vi "max data.vi"() -> (2 "MAX ID":string)   [LabVIEW 2013]
uses:
  <vilib>/addons/database/Connection.llb/DB Tools Open Connec (String).vi
  <vilib>/addons/database/Connection.llb/Conn Execute.vi
  <vilib>/addons/database/Recordset.llb/Rec Fetch Recordset Data (R).vi
  <vilib>/addons/database/Recordset.llb/Rec Destroy - Connection.vi
  <vilib>/addons/database/NI_Database_API.lvlib
panel:
  out "data":string[][](array[string])
  out "recordset data":variant[][](array[variant])
  out "连接的字符串":string
  in  "error in (no error)":errorcluster
  out "error out":errorcluster
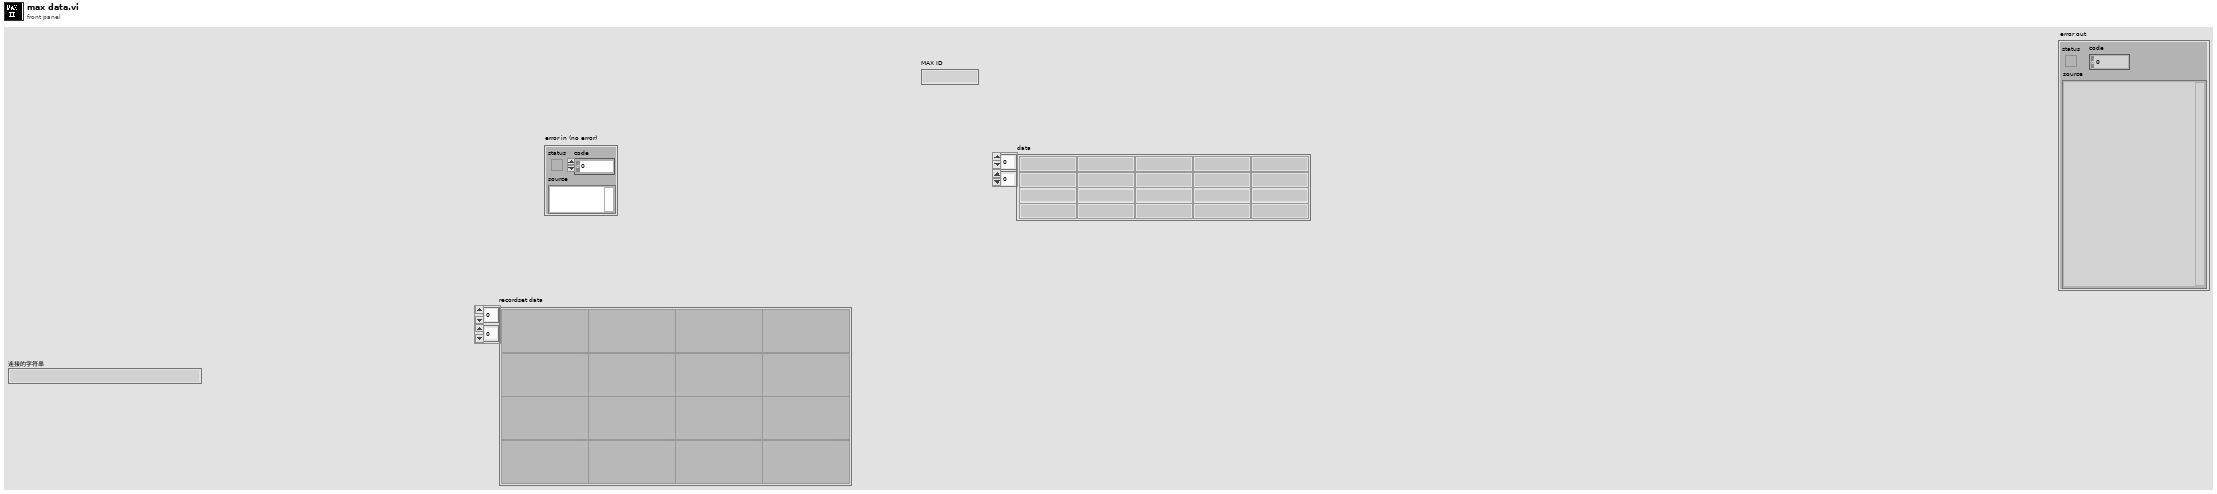
[diagram p1: front panel]
types:
  T1 = typedef "NI_Database_API.lvlib/Conn ObjectReference.ctl" = refnum<k1>
  T2 = typedef "NI_Database_API.lvlib/Rec ObjectReference.ctl" = refnum<k1>
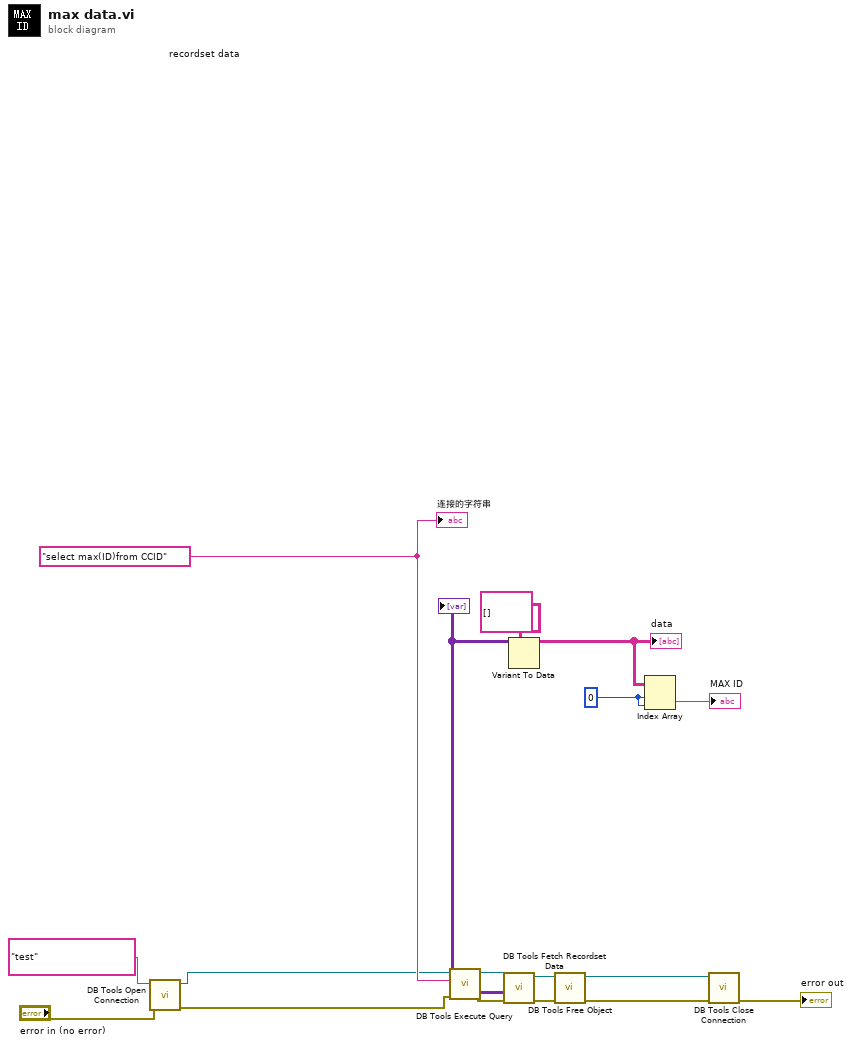
[diagram p0: block diagram]
diagram:
  w2 = 0 ("索引 (行)")
  w6 = "select max(ID)from CCID" ("字符串")
  n1 = call-poly <vilib>:"DB Tools Open Connection.vi"("error in (no error)"="error in (no error)", "connection information"="test" ("userID")) -> ("error out"=w4:errorcluster, "connection reference"=w5:T1)  [unwired: 6 in]
  n2 = call-poly <vilib>:"DB Tools Execute Query.vi"("error in (no error)"=w4, "SQL query"=w6, "connection reference"=w5) -> ("error out"=w14:errorcluster, "recordset reference"=w15:T2)  [unwired: 5 in]
  n3 = call-poly <vilib>:"DB Tools Fetch Recordset Data.vi"("error in (no error)"=w14, "recordset reference"=w15) -> ("error out"=w13:errorcluster, "recordset data"=w10:variant[][], "recordset reference out"=w12:T2)  [unwired: 3 in]
  "recordset data" <- w10
  n4 = Variant To Data(type=string[][] [] ("数组"), Variant=w10) -> (data=w3:string[][])  [unwired: 1 in, 1 out]
  "data" <- w3
  n5 = call-poly <vilib>:"DB Tools Free Object.vi"("error in (no error)"=w13, "recordset reference"=w12) -> ("error out"=w8:errorcluster, "connection reference"=w7:T1)  [unwired: 8 in]
  n6 = Index Array(array=w3, index (row)=w2, index (col)=w2) -> (element=→"MAX ID":string)
  n7 = call <vilib>:"DB Tools Close Connection.vi"("error in (no error)"=w8, "connection reference"=w7) -> ("error out"=→"error out":errorcluster)  [unwired: 5 in]
  "连接的字符串" <- w6
